vi "Update Relation.vi"(8 "error in (no error)":errorcluster, 10 "Relation":refnum<class "Relation.lvclass">, 11 "Entity Editor in":refnum<class "Entity Editor.lvclass">) -> (0 "error out":errorcluster, 3 "Entity Editor out":refnum<class "Entity Editor.lvclass">)   [LabVIEW 2020, in "Conditum-Tools.lvlib" / "Entity Editor.lvclass"]
uses:
  Entity Editor.lvclass
  Conditum-Clone/Columns/Relation/Relation.lvclass
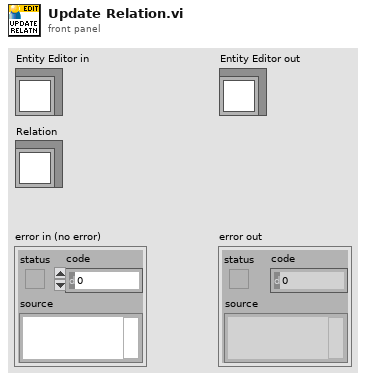
[diagram p1: front panel]
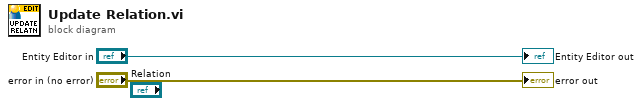
[diagram p0: block diagram]
diagram:
  "error out" <- "error in (no error)"
  "Entity Editor out" <- "Entity Editor in"
